vi "rs3 get Tare status.vi"(7 "error in (no error)":errorcluster, 10 "device in":u64) -> (0 "error out":errorcluster, 1 "error":u64, 3 "Device out":u64, 4 "status":T1(ring))   [LabVIEW 2017, in "libRealSense3.lvlib"]
doc: "Gets the status of tare calibration\n \nparam[in] device RealSense device\nparam[out] error if non-null, receives any error that occurs during this call, otherwise, errors are ignored\n\nreturn the status"
uses:
  libRealSense3.lvlib
  realsense2.dll
panel:
  # "RS3 Get Tare Status"
  # "(C) Intel Corp. 2019,  AGJ"
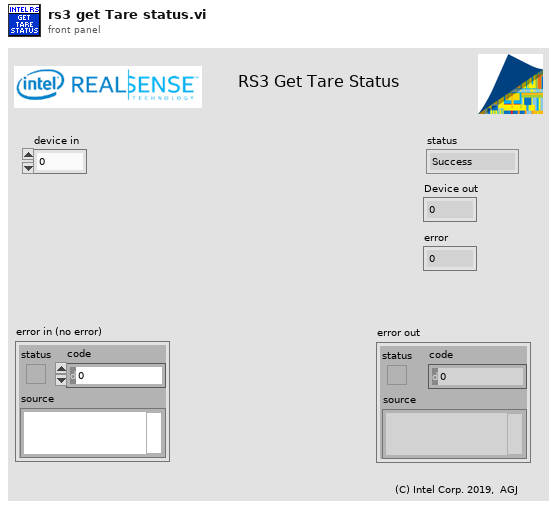
[diagram p1: front panel]
types:
  T1 = enum32{"Success", "Result Not Ready", "Fill factor too low", "Edge too close", "Did not converge"}
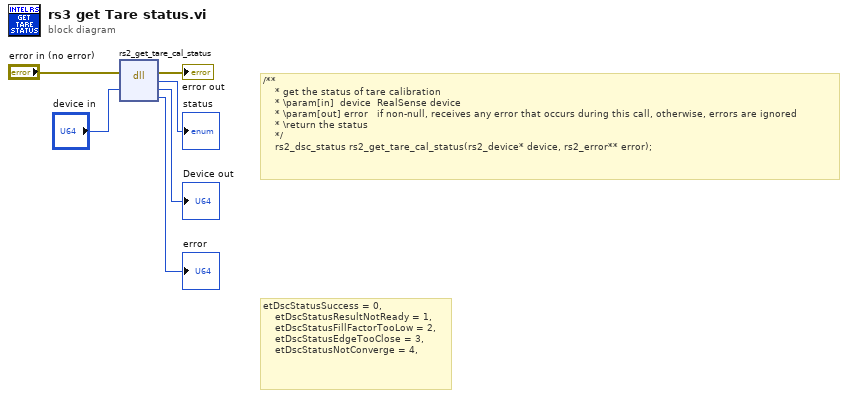
[diagram p0: block diagram]
diagram:
  # "/**\n    * get the status of tare calibration\n    * \\param[in]  device  RealSense device\n    * \\param[out] error   if non-null, receives any error that occurs during this call, otherwise, errors are ignored\n    * \\return the status\n    */\n    rs2_dsc_status rs2_get_tare_cal_status(rs2_device* device, rs2_error** error);"
  # "etDscStatusSuccess = 0,\n    etDscStatusResultNotReady = 1,\n    etDscStatusFillFactorTooLow = 2,\n    etDscStatusEdgeTooClose = 3,\n    etDscStatusNotConverge = 4,"
  n1 = dll-call lib="C:/Users/agrunnet/Documents/libRealSense6/realsense2.dll" fn="rs2_get_tare_cal_status"(error in="error in (no error)", "device"="device in") -> (error out=→"error out":errorcluster, "result"=→"status":i32, "device"=→"Device out":u64, "error"=→"error":u64)  [unwired: 3 in, 1 out]
